vi "RomanToInteger.vi"(8 "error in (no error)":errorcluster, 11 "String":string) -> (0 "error out":errorcluster, 3 "Numeric":i32)   [LabVIEW 2023]
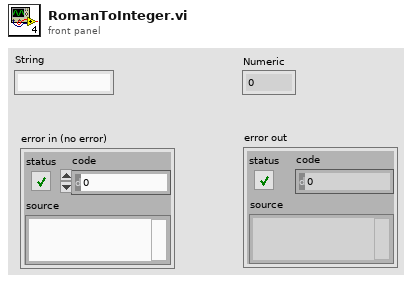
[diagram p1: front panel]
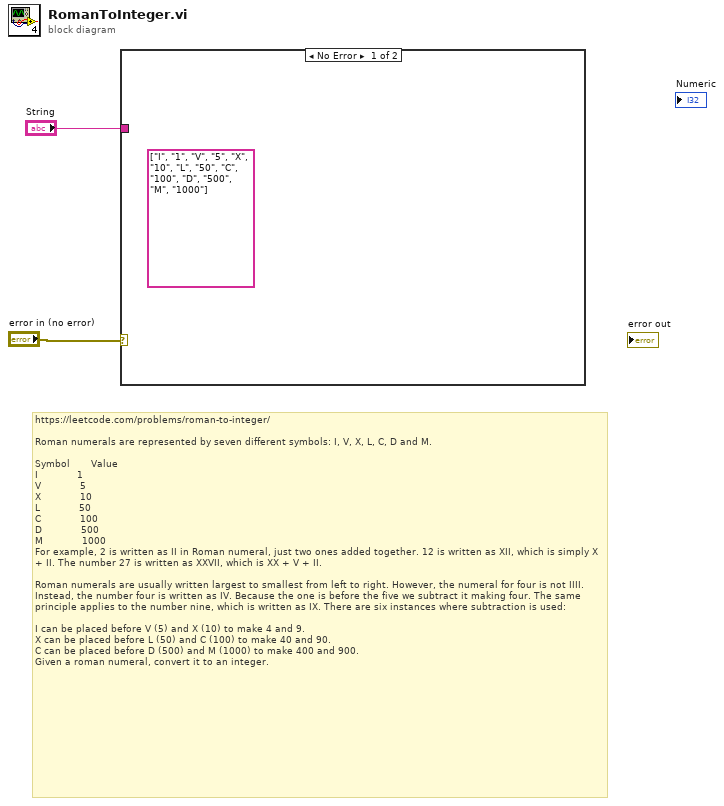
[diagram p0: block diagram]
diagram:
  # "https://leetcode.com/problems/roman-to-integer/\n\nRoman numerals are represented by seven different symbols: I, V, X, L, C, D and M.\n\nSymbol       Value\nI             1\nV             5\nX             10\nL             50\nC             100\nD             500\nM             1000\nFor example, 2 is written as II in Roman numeral, just two ones added together. 12 is written as XII, which is simply X + II. The number 27 is written as XXVII, which is XX + V + II.\n\nRoman numerals are usually written largest to smallest from left to right. However, the numeral for four is not IIII. Instead, the number four is written as IV. Because the one is before the five we subtract it making four. The same principle applies to the number nine, which is written as IX. There are six instances where subtraction is used:\n\nI can be placed before V (5) and X (10) to make 4 and 9. \nX can be placed before L (50) and C (100) to make 40 and 90. \nC can be placed before D (500) and M (1000) to make 400 and 900.\nGiven a roman numeral, convert it to an integer."
  n1 = case shown="No Error" "error in (no error)" {
    tunnel: "String" -> [_ _]
    frame No Error {
      (unwired) string[][] [["I", "1"], ["V", "5"], ["X", "10"], ["L", "50"], ["C", "100"], ["D", "500"], ["M", "1000"]]
    }
    frame Error {
    }
  }
